vi "GFITS_LibSetRoi.vi"(4 "ylen":u32, 5 "ystart":u32, 6 "xlen":u32, 7 "xstart":u32, 8 "error in (no error)":errorcluster) -> (0 "error IO":errorcluster, 3 "return type":i32)   [LabVIEW 2016]
uses:
  c/lib/libgfits.so
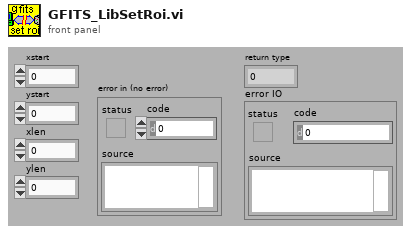
[diagram p1: front panel]
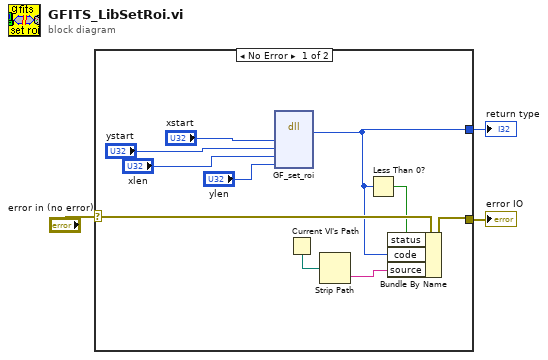
[diagram p0: block diagram]
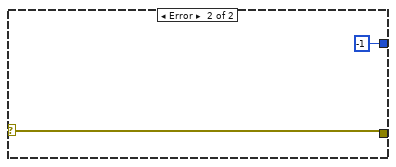
[diagram p2: hidden frame]
diagram:
  n1 = case shown="No Error" "error in (no error)" {
    selector: "error in (no error)" -> [w13 w15]
    tunnel: [w11 -1 ("return type")] -> w2
    tunnel: [w8 w15] -> w1
    frame No Error {
      n2 = dll-call lib="home/simager/panview/PAN/Modules/GFITS/private/c/lib/libgfits.so" fn="GF_set_roi"("xstart"="xstart", "ystart"="ystart", "xlen"="xlen", "ylen"="ylen") -> ("return type"=w11:i32)  [unwired: 7 in, 2 out]
      n3 = Current VI's Path() -> (path=w10:path)
      n4 = Strip Path(path=w10) -> (name=w9:string)  [unwired: 1 out]
      n5 = Less Than 0?(x=w11) -> (x < 0?=w12:bool)
      n6 = Bundle By Name(cluster=w13, "status"=w12, "code"=w11, "source"=w9) -> (w8:errorcluster)
    }
    frame Error {
    }
  }
  "return type" <- w2
  "error IO" <- w1
